vi "bye.vi"(8 "error in (no error)":errorcluster, 11 "simonMessages in":refnum<class "simonMessages.lvclass">) -> (0 "error out":errorcluster, 3 "simonMessages out":refnum<class "simonMessages.lvclass">)   [LabVIEW 2020, in "simonMessages.lvclass"]
uses:
  simonMessages.lvclass
  simonMessages.lvclass/simonMessages.ctl
  TextDisplay/TextDisplay Class.lvclass
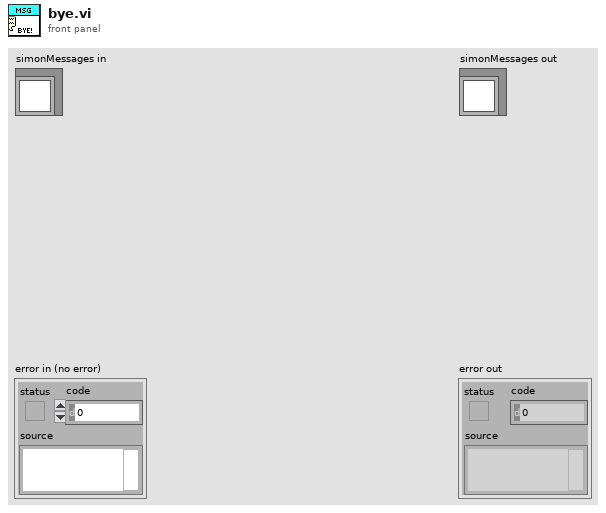
[diagram p1: front panel]
types:
  T1 = cluster{"Text":string, "Size":u8, "Justification":enum16{"Left", "Center", "Right"}, "Display Type":string}
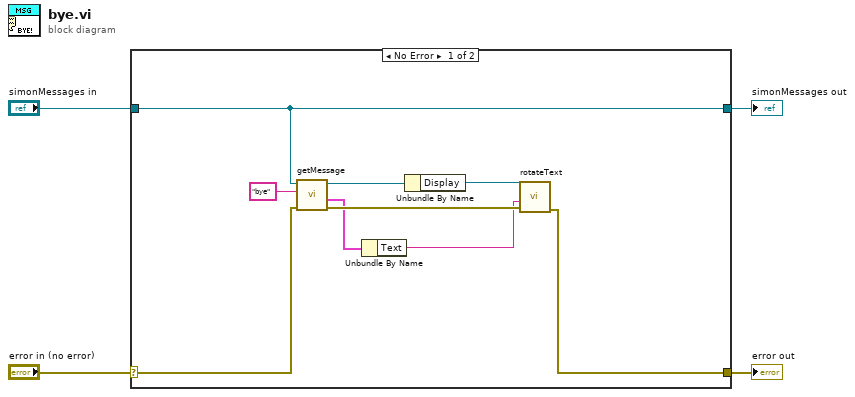
[diagram p0: block diagram]
diagram:
  n1 = case shown="No Error" "error in (no error)" {
    selector: "error in (no error)" -> [w8 w15]
    tunnel: [w7 w15] -> w3
    tunnel: [w10 w14] -> w1
    tunnel: "simonMessages in" -> [w10 w14]
    frame No Error {
      n2 = call "getMessage.vi"("error in (no error)"=w8, "key"="bye", "simonMessages in"=w10) -> ("error out"=w9:errorcluster, "Message Cluster"=w6:T1, "simonMessages out"=w13:refnum<class "simonMessages.lvclass">)  [unwired: 6 in]
      n3 = Unbundle By Name(w6) -> ("Text"=w5:string)
      n4 = Unbundle By Name(w13) -> ("Display"=w11:refnum<class "TextDisplay Class.lvclass">)
      n5 = call "rotateText.vi"("error in (no error)"=w9, "textIn"=w5, "TextDisplay Class in"=w11) -> ("error out"=w7:errorcluster)  [unwired: 7 in, 1 out]
    }
    frame Error {
    }
  }
  "error out" <- w3
  "simonMessages out" <- w1
